vi "_Lookup Channel.vi"(8 "error in (no error)":errorcluster, 10 "Channel Name":string, 11 "Loop Data in":T1) -> (0 "error out":errorcluster, 2 "Channel":refnum<class "Channel.lvclass">, 3 "Loop Data":T1)   [LabVIEW 2020, in "Vecto.lvlib" / "ChannelService.lvclass"]
uses:
  ChannelService.lvclass
  Loop Data.ctl
  Group/Group.lvclass
  Channel/Channel.lvclass
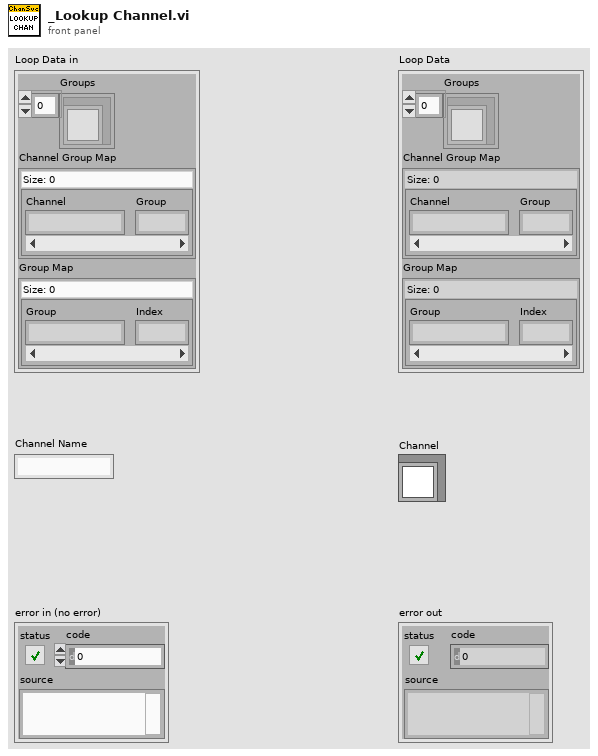
[diagram p1: front panel]
types:
  T1 = typedef "Vecto.lvlib/ChannelService.lvclass/Loop Data.ctl" = cluster{"Groups":refnum<class "Group.lvclass">[], "Channel Group Map":map{string, i32}, "Group Map":map{string, i32}}
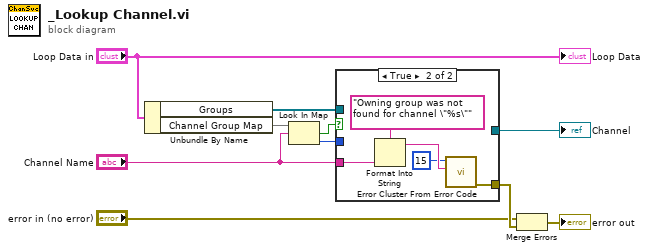
[diagram p0: block diagram]
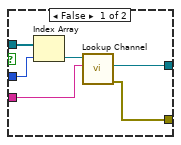
[diagram p2: hidden frame]
diagram:
  n1 = Unbundle By Name("Loop Data in") -> ("Groups"=w7:refnum<class "Group.lvclass">[], "Channel Group Map"=w10:map{string, i32})
  n2 = Look In Map(map=w10, key="Channel Name") -> (key not found?=w9:bool, value=w8:i32)  [unwired: 1 in]
  n3 = case shown="True" w9 {
    tunnel: w8 -> [w15 _]
    tunnel: w7 -> [w16 _]
    tunnel: "Channel Name" -> [w13 w21]
    tunnel: [w12 _] -> w4
    tunnel: [w11 w17] -> w3
    frame False {
      n4 = Index Array(array=w16, index=w15) -> (element=w14:refnum<class "Group.lvclass">)
      n5 = call "Lookup Channel.vi"("Channel Name"=w13, "Group in"=w14) -> ("error out"=w11:errorcluster, "Channel"=w12:refnum<class "Channel.lvclass">)  [unwired: 7 in, 1 out]
    }
    frame True {
      n6 = Format Into String(format string="Owning group was not found for channel \"%s\"", w21) -> (resulting string=w19:string)  [unwired: 2 in, 1 out]
      n7 = call <vilib>:"Error Cluster From Error Code.vi"("error message (\"\")"=w19, "error code (0)"=15) -> ("error out"=w17:errorcluster)  [unwired: 7 in]
    }
  }
  "Channel" <- w4
  n8 = Merge Errors("error in (no error)", w3) -> (→"error out":errorcluster)
  "Loop Data" <- "Loop Data in"
